vi "FTP2WEB Worker RD v1.0 (SubVI).vi"(4 "FTP Remote Path":string, 5 "FTP Password":string, 6 "FTP Host":string, 7 "FTP Username":string="anonymous", 8 "error in (no error)":errorcluster, 9 "Temp Filename":string, 10 "Local File Path":string, 11 "FTP Delete After Upload?":bool) -> (0 "error out":errorcluster)   [LabVIEW 2019]
doc: "FTP Worker Core. \n\n2019 NREL"
uses:
  Globals and Definitions/Initialization Globals.vi
  <vilib>/FTP/NI_FTP.lvlib
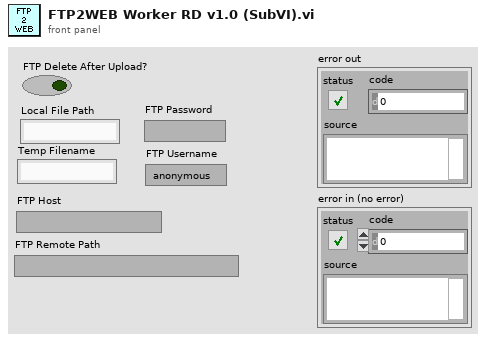
[diagram p1: front panel]
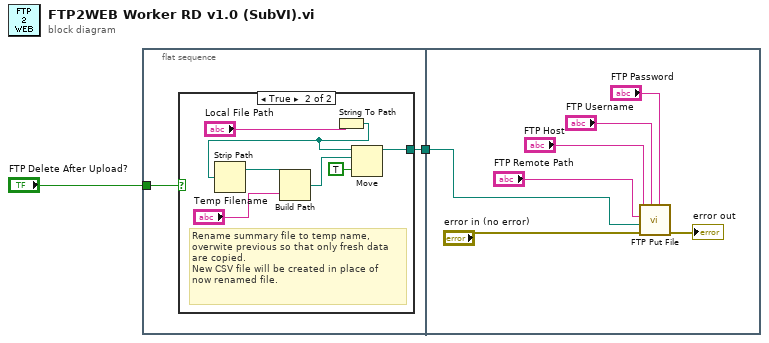
[diagram p0: block diagram]
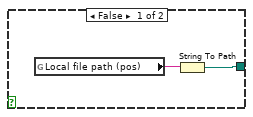
[diagram p2: hidden frame]
diagram:
  n1 = flat-sequence {
    tunnel: [w4] -> w2
    tunnel: "FTP Delete After Upload?" -> [w3]
    tunnel: w2 -> [w18]
    frame #0 {
      n2 = case shown="True" w3 {
        tunnel: [w5 w10] -> w4
        frame False {
          n3 = global read "Initialization Globals.vi" "Local file path (pos)"() -> (w6:string)
          n4 = String To Path(string=w6) -> (path=w5:path)
        }
        frame True {
          # "Rename summary file to temp name,\noverwite previous so that only fresh data\nare copied. \nNew CSV file will be created in place of \nnow renamed file."
          # "Rename summary file"
          n5 = String To Path(string="Local File Path") -> (path=w9:path)
          n6 = Strip Path(path=w9) -> (stripped path=w12:path)  [unwired: 1 out]
          n7 = Build Path(base path=w12, name or relative path="Temp Filename") -> (appended path=w13:path)
          n8 = Move(source path=w9, 9:TRUE ("overwrite (F)"), 10:w13) -> (3:w10:path)  [unwired: 2 in, 2 out]
        }
      }
    }
    frame #1 {
      n9 = call <vilib>:"FTP Put File.vi"("password"="FTP Password", "user"="FTP Username", "error in (no error)"="error in (no error)", "local path"=w18, "remote path"="FTP Remote Path", "host"="FTP Host") -> ("error out"=→"error out":errorcluster)  [unwired: 4 in, 1 out]
    }
  }
